vi "ObtainRequestEvents.vi"(8 "Error":errorcluster[](array[cluster])) -> (0 "Error":errorcluster[](array[cluster]), 3 "clRequestEvents":T1)   [LabVIEW 2014, in "Visualization.lvlib" / "VisualizeFlags.lvclass"]
uses:
  VisualizeFlags.lvclass
  VisializeBase_class/Requests/clUserEventType.ctl
  VisializeBase_class/VisualizeBase_class.lvclass
  <userlib>/NIST/NISTErrorLib/NISTErrorLib.lvlib
  VisializeBase_class/Requests/clRequestEvents.ctl
panel:
  # "If you want to add other Request Events, open this typedef, copy an existing event and rename it to your event name."
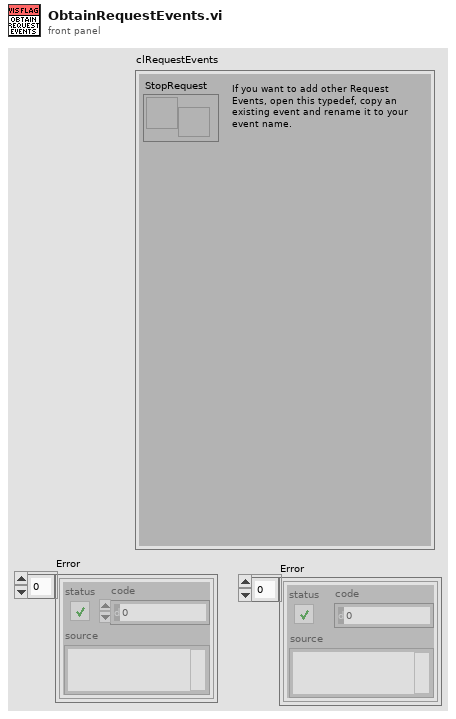
[diagram p1: front panel]
types:
  T1 = typedef "Visualization.lvlib/VisualizeBase_class.lvclass/clRequestEvents.ctl" = cluster{"StopRequest":refnum<user-event>}
  T2 = typedef "Visualization.lvlib/clRequestEvents.ctl" = cluster{"StopRequest":refnum<user-event>}
  T3 = typedef "Visualization.lvlib/VisualizeBase_class.lvclass/clUserEventType.ctl" = cluster{"BusIndex":i8, "Data":variant}
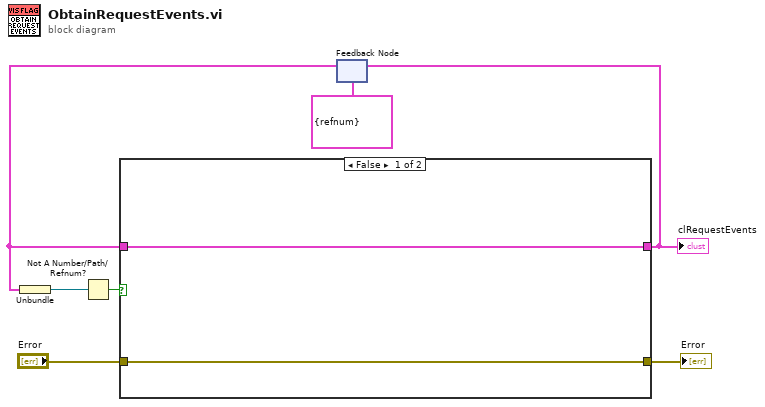
[diagram p0: block diagram]
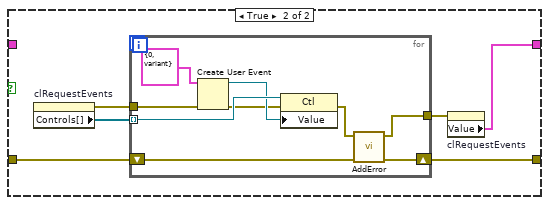
[diagram p2: hidden frame]
diagram:
  n1 = feedback #1(T1 {"StopRequest"=refnum} ("Value")) -> (w3:T2)
  n2 = Unbundle(w3) -> ("StopRequest"=w1:refnum<user-event>)
  n3 = Not A Number/Path/Refnum?(number/path/refnum=w1) -> (NaN/Path/Refnum?=w2:bool)
  n4 = case shown="False" w2 {
    tunnel: [w9 w10] -> w7
    tunnel: w3 -> [w9 _]
    tunnel: [w8 w12] -> w5
    tunnel: "Error" -> [w8 w13]
    frame False {
    }
    frame True {
      n5 = property on="clRequestEvents" class="Clust (strict)"() -> (error out=w14:errorcluster, "Controls[]"=w15:refnum<vi>[])  [unwired: 2 in, 1 out]
      n6 = for {
        tunnel: w15 -> [w22] mode=indexing
        tunnel: w14 -> [w23]
        shift-right: [w17] -> w12
        shift-left: w13 -> [w18]
        tunnel: [w16] -> w11
        n7 = Create User Event(user event datatype=T3 {"BusIndex"=0, "Data"=variant} ("clEventType"), error in=w23) -> (user event=w21:refnum<user-event>, error out=w20:errorcluster)
        n8 = property class="Ctl"(reference=w22, error in=w20, "Value"=w21) -> (error out=w19:errorcluster)  [unwired: 1 out]
        n9 = call <userlib>:"AddError.vi"("ErrorArray"=w18, "error in (no error)"=w19) -> ("ErrorArray"=w17:errorcluster[], "error out"=w16:errorcluster)  [unwired: 8 in]
      }
      n10 = property on="clRequestEvents" class="Clust (strict)"(error in=w11) -> ("Value"=w10:T2)  [unwired: 1 in, 2 out]
    }
  }
  "clRequestEvents" <- w7
  "Error" <- w5
  n11 = feedback-in #1(w7) -> ()
